vi "Gyro Recalibrate Loop.vi"   [LabVIEW 2013]
uses:
  <vilib>/Rock Robotics/SystemInterfaces/AI/FPGA_AIGyroChannel.ctl
  Robot Global Data.vi
types:
  T1 = typedef "FPGA_AIGyroChannel.ctl" = enum8{"AI 1", "AI 2", "Invalid"}
  T2 = typedef "WPI_GyroDevRef.ctl" = cluster{"DevStatus":errorcluster, "Analog Module":T3, "Analog Channel":T4, "Offset":dbl, "Gain (VoltsPerDegree/Second)":dbl}
  T3 = typedef "FPGA_TypedefAnalogModule.ctl" = enum16{"Analog Module 1", "Analog Module 2"}
  T4 = typedef "FPGA_AIChannel.ctl" = enum8{"AI 1", "AI 2", "AI 3", "AI 4", "AI 5", "AI 6", "AI 7", "AI 8", "Invalid"}
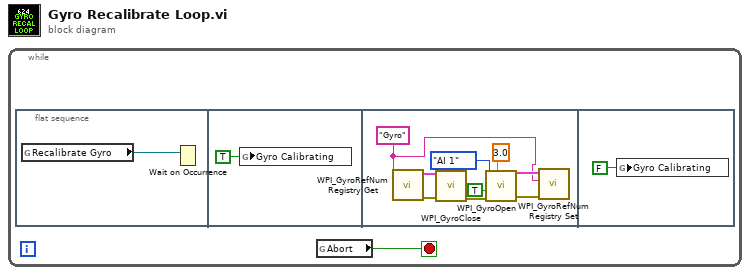
[diagram p0: block diagram]
diagram:
  n1 = while {
    stop <- w1 stop-if-true
    n2 = flat-sequence {
      frame #0 {
        n3 = global read "Robot Global Data.vi" "Recalibrate Gyro"() -> (w2:refnum<k4>)
        n4 = Wait on Occurrence(2:w2) -> ()  [unwired: 2 in, 1 out]
      }
      frame #1 {
        n5 = global write "Robot Global Data.vi" "Gyro Calibrating"(TRUE) -> ()
      }
      frame #2 {
        w4 = "Gyro" ("refnum name")
        n6 = call <vilib>:"WPI_GyroRefNum Registry Get.vi"("refnum name"=w4) -> ("error out"=w12:errorcluster, "GyroDevRef"=w11:T2)  [unwired: 9 in]
        n7 = call <vilib>:"WPI_GyroClose.vi"("error in (no error)"=w12, "GyroDevRef"=w11) -> ("error out"=w10:errorcluster)  [unwired: 9 in]
        n8 = call <vilib>:"WPI_GyroOpen.vi"("Calibration Time (s)"=3.0, "error in (no error)"=w10, "Calibrate On Open"=TRUE, "Analog Channel"=FPGA_AIGyroChannel."AI 1") -> ("error out"=w6:errorcluster, "GyroDevRef"=w5:T2)  [unwired: 5 in, 1 out]
        n9 = call <vilib>:"WPI_GyroRefNum Registry Set.vi"("error in (no error)"=w6, "refnum name"=w4, "GyroDevRef"=w5) -> ()  [unwired: 7 in, 2 out]
      }
      frame #3 {
        n10 = global write "Robot Global Data.vi" "Gyro Calibrating"(FALSE) -> ()
      }
    }
    n11 = global read "Robot Global Data.vi" "Abort"() -> (w1:bool)
  }
